vi "Create_and_save_to_file (SubVI).vi"(1 "Место сохранения":path, 2 "input string":string, 3 "error in":errorcluster) -> (6 "Текущее расположение файла":path, 7 "error out":errorcluster)   [LabVIEW 8.6]
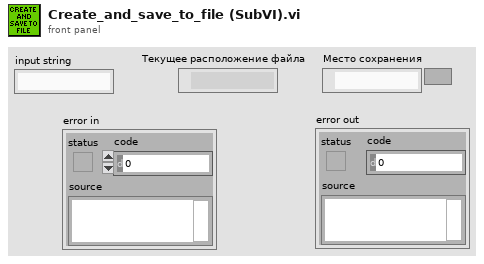
[diagram p1: front panel]
types:
  T1 = enum16{"open", "replace", "create", "open or create", "replace or create", "replace or create with confirmation"}
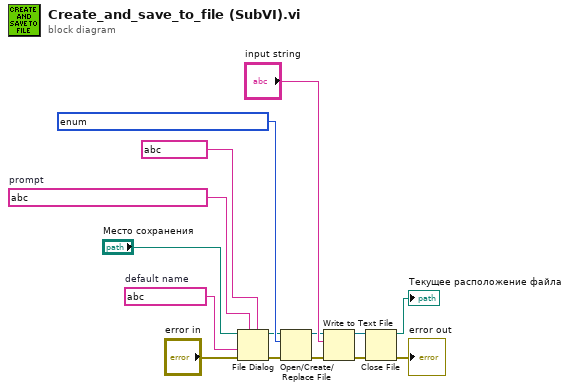
[diagram p0: block diagram]
diagram:
  w12 = string ?  # default name
  w11 = string ?  # prompt
  n1 = File Dialog(5:string ? ("button label"), 7:w11, 8:"error in", 9:w12, 11:"Место сохранения") -> (0:w13:errorcluster, 3:w5:path)  [unwired: 4 out]
  n2 = Open/Create/Replace File(file path (use dialog)=w5, error in=w13, operation (0:open)=T1 ?) -> (refnum out=w7:refnum<file>, error out=w10:errorcluster)  [unwired: 4 out]
  n3 = Write to Text File(file (use dialog)=w7, text="input string", error in=w10) -> (refnum out=w2:refnum<file>, error out=w4:errorcluster)  [unwired: 2 out]
  n4 = Close File(refnum=w2, error in=w4) -> (path=→"Текущее расположение файла":path, error out=→"error out":errorcluster)
